vi "Large integer U8 array - fast modular exp.vi"(9 "n (LI_U8)":T1=[177, 202, 163, 228, 80, 172, 92, 0, 203, 107, 235, 193], 10 "Exponent e (LI-U8)":T1=[88, 229, 81, 114, 40, 86, 46, 128, 229, 181, 245, 96], 11 "B (LI-U8)":T1=[143, 6, 191, 254, 56, 141, 240, 118, 65, 169, 219]) -> (1 "iterations":u32=94, 3 "B^e mod n":T1=[176, 202, 163, 228, 80, 172, 92, 0, 203, 107, 235, 193])   [LabVIEW 2013]
doc: "Uses a fast modular exponential algorithm to calculate B^e mod n (remainder after dividing B^e by n)."
uses:
  User Access Type defs/Large number - U8 array.ctl
panel:
  out "current iteration":i32=4
  # "Johnson example\nB = 4183\ne = 17143\nn = 60491\nBe mod n = 436"
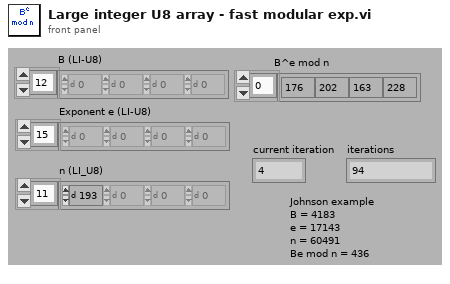
[diagram p1: front panel]
types:
  T1 = typedef "Large number - U8 array.ctl" = u8[]
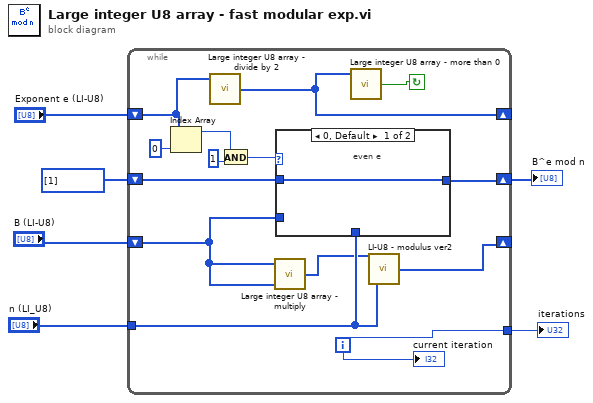
[diagram p0: block diagram]
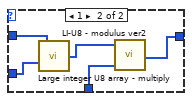
[diagram p2: hidden frame]
diagram:
  n1 = while {
    shift-right: [w16] -> _
    shift-left: "Exponent e (LI-U8)" -> [w17]
    shift-right: [w12] -> w3
    shift-left: T1 [1] ("Large number -U8 B") -> [w13]
    shift-right: [w8] -> _
    shift-left: "B (LI-U8)" -> [w11]
    tunnel: "n (LI_U8)" -> [w9]
    tunnel: [w10] -> w1
    i -> [w10]
    stop <- w15 continue-if-true
    n2 = Index Array(array=w17, index=0) -> (element=w18:u8)
    n3 = call "Large integer U8 array - divide by 2.vi"("Large number - U8"=w17) -> ("Divided by 2"=w16:T1)  [unwired: 4 out]
    n4 = And(x=w18, y=u32 1) -> (x .and. y?=w14:u32)
    n5 = call "Large integer U8 array - multiply.vi"("Large number - U8 2"=w11, "Large number - U8 1"=w11) -> ("Multiplied array"=w7:T1)  [unwired: 3 out]
    n6 = case shown="0, Default" w14 {
      tunnel: [w21 w22] -> w12
      tunnel: w13 -> [w21 w26]
      tunnel: w11 -> [_ w25]
      tunnel: w9 -> [_ w23]
      frame 0, Default {
        # "even e"
      }
      frame 1 {
        n7 = call "Large integer U8 array - multiply.vi"("Large number - U8 2"=w25, "Large number - U8 1"=w26) -> ("Multiplied array"=w24:T1)  [unwired: 3 out]
        n8 = call "LI-U8 - modulus ver2.vi"("Large number - U8 B"=w23, "Large number - U8 A"=w24) -> ("A mod (B)"=w22:T1)  [unwired: 3 out]
      }
    }
    n9 = call "Large integer U8 array - more than 0.vi"("Large number - U8"=w16) -> ("> 0 ?"=w15:bool)  [unwired: 4 out]
    n10 = call "LI-U8 - modulus ver2.vi"("Large number - U8 B"=w9, "Large number - U8 A"=w7) -> ("A mod (B)"=w8:T1)  [unwired: 3 out]
    "current iteration" <- w10
  }
  "B^e mod n" <- w3
  "iterations" <- w1
